vi "NTV_Drive CMD Data.vi"(7 "Read(f) Write(t)":bool, 11 "Comand Data":T1 {"Rotate(Yaw) CCW 1 CW -1" scale=1.0..-1.0; "Traverse"."Angle" scale format="%.3f"; "Traverse"."Velocity" scale=-1.0..1.0 scale format="%.1f"}) -> (3 "Comand Data Out":T1 {"Rotate(Yaw) CCW 1 CW -1" scale=1.0..-1.0; "Traverse"."Angle" scale format="%.3f"; "Traverse"."Velocity" scale=-1.0..1.0 scale format="%.1f"})   [LabVIEW 2023]
uses:
  TypeDefs/Cluster_CMD_Direction Data.ctl
  TypeDefs/Cluster_Module Velocity-Direction-Rotations.ctl
  TypeDefs/Level_Velocity plus-minus 1.ctl
  TypeDefs/Dial_Compase heading unit circle CCW positive.ctl
  <vilib>/Rock Robotics/Network Tables/NT Read Numeric Array.vi
  <vilib>/Rock Robotics/Network Tables/NT Write Numeric Array.vi
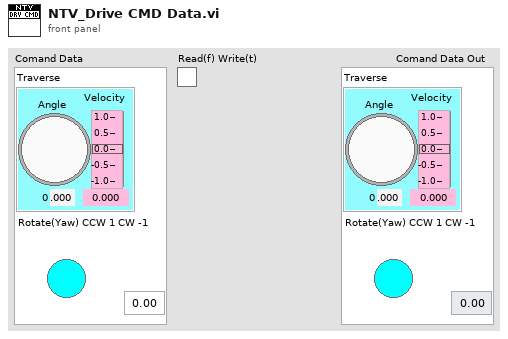
[diagram p1: front panel]
types:
  T1 = typedef "Cluster_CMD_Direction Data.ctl" = cluster{"Traverse":T2, "Rotate(Yaw) CCW 1 CW -1":dbl}
  T2 = typedef "Cluster_Module Velocity-Direction-Rotations.ctl" = cluster{"Velocity":T3, "Angle":T4, "Rotations Count":dbl}
  T3 = typedef "Level_Velocity plus-minus 1.ctl" = dbl
  T4 = typedef "Dial_Compase heading unit circle CCW positive.ctl" = dbl
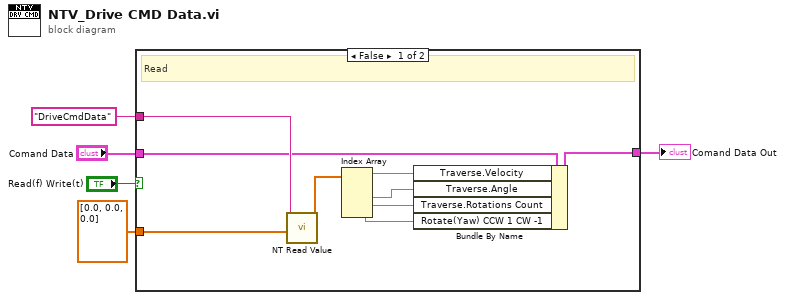
[diagram p0: block diagram]
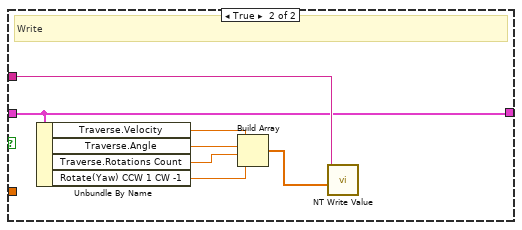
[diagram p2: hidden frame]
diagram:
  n1 = case shown="False" "Read(f) Write(t)" {
    tunnel: "Comand Data" -> [w12 w20]
    tunnel: "DriveCmdData" ("Name") -> [w14 w21]
    tunnel: [w11 w20] -> w1
    tunnel: dbl[] [0.0, 0.0, 0.0] ("Default Value") -> [w13 _]
    frame False {
      # "Read"
      n2 = call-poly <vilib>:"NT Read Value.vi"("default value"=w13, "name"=w14) -> ("value"=w10:dbl[])  [unwired: 7 in, 2 out]
      n3 = Index Array(array=w10) -> (element #1=w9:dbl, element #2=w8:dbl, element #3=w7:dbl, element #4=w6:dbl)  [unwired: 4 in]
      n4 = Bundle By Name(cluster=w12, "Traverse.Velocity"=w9, "Traverse.Angle"=w8, "Traverse.Rotations Count"=w7, "Rotate(Yaw) CCW 1 CW -1"=w6) -> (w11:T1)
    }
    frame True {
      # "Write"
      n5 = Unbundle By Name(w20) -> ("Traverse.Velocity"=w17:T3, "Traverse.Angle"=w19:T4, "Traverse.Rotations Count"=w18:dbl, "Rotate(Yaw) CCW 1 CW -1"=w16:dbl)
      n6 = Build Array(w17, w19, w18, w16) -> (w15:T4[])
      n7 = call-poly <vilib>:"NT Write Value.vi"("value"=w15, "name"=w21) -> ()  [unwired: 9 in, 1 out]
    }
  }
  "Comand Data Out" <- w1
